vi "FT_Get_Status_64bit.vi"(0 "Handle":u64, 11 "error in (no error)":errorcluster) -> (4 "Handle out":u64, 6 "FT_Status":u32(ring) items=["FT_OK", "FT_INVALID_HANDLE", "FT_DEVICE_NOT_FOUND", "FT_DEVICE_NOT_OPENED", "FT_IO_ERROR", "FT_INSUFFICIENT_RESOURCES", "FT_INVALID_PARAMETER", "FT_INVALID_BAUD_RATE", "FT_DEVICE_NOT_OPENED_FOR_ERASE", "FT_DEVICE_NOT_OPENED_FOR_WRITE", "FT_FAILED_TO_WRITE_DEVICE", "FT_EEPROM_READ_FAILED", "FT_EEPROM_WRITE_FAILED", "FT_EEPROM_ERASE_FAILED", "FT_EEPROM_NOT_PRESENT", "FT_EEPROM_NOT_PROGRAMMED", "FT_INVALID_ARGS", "FT_NOT_SUPPORTED", "FT_OTHER_ERROR"], 8 "Event Status":u32(ring) items=["None", "FT_EVENT_RXCHAR", "FT_EVENT_MODEM_STATUS"], 12 "RX Bytes":u32, 14 "TX Bytes":u32, 15 "error out":errorcluster)   [LabVIEW 2019]
uses:
  FTD2XX.dll
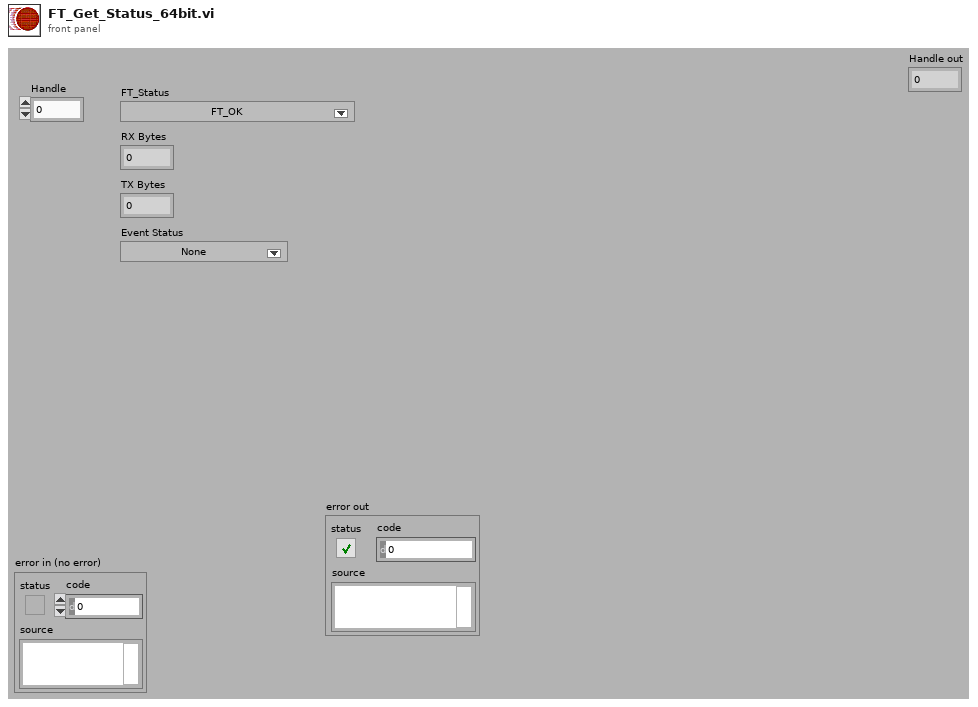
[diagram p1: front panel]
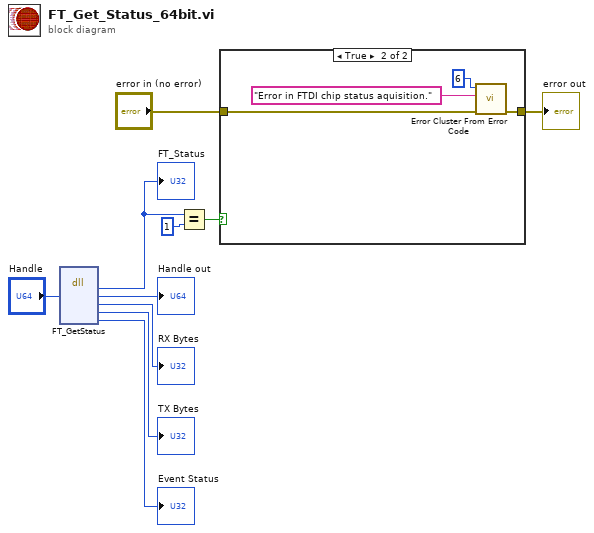
[diagram p0: block diagram]
diagram:
  n1 = dll-call lib="ftd2xx.dll" fn="FT_GetStatus"("Handle"="Handle") -> ("FT_Status"=w1:u32, "Handle"=→"Handle out":u64, "AmountInRxQueue"=→"RX Bytes":u32, "AmountInTxQueue"=→"TX Bytes":u32, "EventStatus"=→"Event Status":u32)  [unwired: 6 in, 2 out]
  "FT_Status" <- w1
  n2 = Equal?(x=w1, y=u32 1) -> (x = y?=w5:bool)
  n3 = case shown="True" w5 {
    tunnel: [w11 w14] -> w2
    tunnel: "error in (no error)" -> [w11 w13]
    frame False {
    }
    frame True {
      n4 = call <vilib>:"Error Cluster From Error Code.vi"("error in (no error)"=w13, "error message (\"\")"="Error in FTDI chip status aquisition." ("error message (\"\")"), "error code (0)"=6) -> ("error out"=w14:errorcluster)  [unwired: 6 in]
    }
  }
  "error out" <- w2
